vi "Workspace.Channels.Create.vi"(11 "CD Path":string) -> (2 "Read Channels":string[](array[string]), 3 "Write Channels":string[](array[string]))   [LabVIEW 2015, in "Diagnostics Addon Shared.lvlib"]
uses:
  Diagnostics Addon Shared.lvlib
  Constants.vi
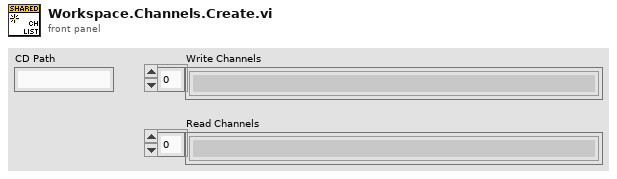
[diagram p1: front panel]
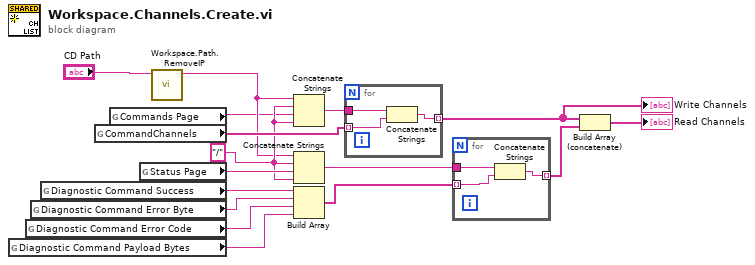
[diagram p0: block diagram]
diagram:
  w5 = "/" ("string")
  n1 = global read "Constants.vi" "Diagnostic Command Payload Bytes"() -> (w14:string)
  n2 = global read "Constants.vi" "Diagnostic Command Error Code"() -> (w13:string)
  n3 = global read "Constants.vi" "Diagnostic Command Error Byte"() -> (w12:string)
  n4 = global read "Constants.vi" "Diagnostic Command Success"() -> (w11:string)
  n5 = global read "Constants.vi" "CommandChannels"() -> (w7:string[])
  n6 = global read "Constants.vi" "Commands Page"() -> (w1:string)
  n7 = global read "Constants.vi" "Status Page"() -> (w8:string)
  n8 = call "Workspace.Path.RemoveIP.vi"("CD Path"="CD Path") -> ("Path"=w3:string)  [unwired: 9 in, 1 out]
  n9 = Concatenate Strings(w3, w5, w1, w5) -> (w6:string)
  n10 = Concatenate Strings(w3, w5, w8, w5) -> (w9:string)
  n11 = Build Array(w11, w12, w13, w14) -> (w15:string[])
  n12 = for {
    tunnel: w6 -> [w19]
    tunnel: w7 -> [w17] mode=indexing
    tunnel: [w18] -> w16 mode=indexing
    n13 = Concatenate Strings(w19, w17) -> (w18:string)
  }
  "Write Channels" <- w16
  n14 = for {
    tunnel: w9 -> [w22]
    tunnel: w15 -> [w20] mode=indexing
    tunnel: [w21] -> w10 mode=indexing
    n15 = Concatenate Strings(w22, w20) -> (w21:string)
  }
  n16 = Build Array (concatenate)(w16, w10) -> (→"Read Channels":string[])
